vi "启动命令国标转换.vi"(11 "启动命令":T2 caption="00：00" items=["", "加标回收（启动采配水）", "加标回收（不启动采配水）", "水样测试（启动采配水）", "水样测试（不启动采配水）"]) -> (3 "控制命令":T1)   [LabVIEW 2016, in "ZK定时设置.xctl"]
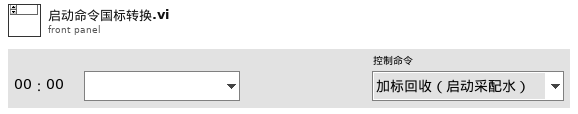
[diagram p1: front panel]
types:
  T1 = typedef "ZK定时设置.xctl/国标控制命令.ctl" = enum16{"加标回收（启动采配水）", "加标回收（不启动采配水）", "水样测试（启动采配水）", "水样测试（不启动采配水）"}
  T2 = typedef "ZK定时设置.xctl/启动命令选择.ctl" = u16
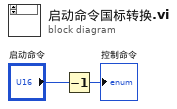
[diagram p0: block diagram]
diagram:
  n1 = Decrement(x="启动命令") -> (x-1=→"控制命令":T2)
